vi "Build Spec Param to XPath.vi"(0 "NI Build Specification":refnum<class "NI Build Specification_LV.lvclass">, 5 "Build Spec Parameter Name":string, 11 "error in (no error)":errorcluster) -> (4 "NI Build Specification":refnum<class "NI Build Specification_LV.lvclass">, 6 "XPath to the specific build Spec Property":string, 15 "error out":errorcluster)   [LabVIEW 2017, in "CL_G3_VIComponentBuilder.lvlib" / "NI Build Specification_LV.lvclass"]
doc: "Returns an Xpath to the parameter of a build specification."
uses:
  NI Build Specification_LV.lvclass
  NI Build Specification_LV.lvclass/NI Build Specification_LV.ctl
  Accessors/Read Target Name Containing Build Specs to Build.vi
  Accessors/Read Export's Build Spec Name.vi
  Accessors/Read Build Spec Type.vi
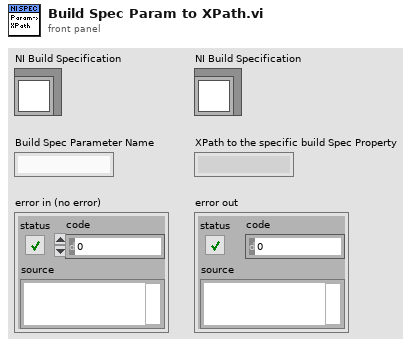
[diagram p1: front panel]
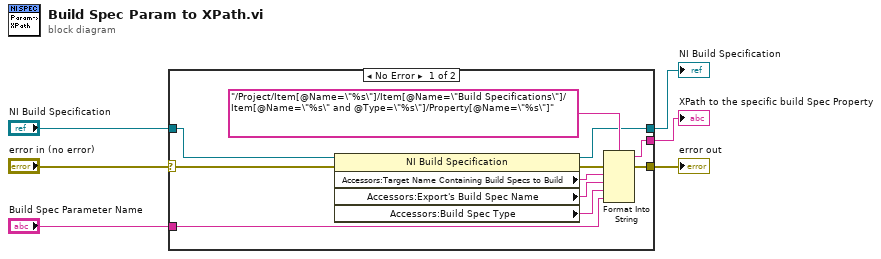
[diagram p0: block diagram]
diagram:
  n1 = case shown="No Error" "error in (no error)" {
    selector: "error in (no error)" -> [w8 w18]
    tunnel: "NI Build Specification" -> [w17 w19]
    tunnel: [w15 w19] -> w5
    tunnel: [w11 _] -> w4
    tunnel: "Build Spec Parameter Name" -> [w9 _]
    tunnel: [w7 w18] -> w1
    frame No Error {
      n2 = property class="NI Build Specification"(reference=w17, error in=w8) -> (reference out=w15:refnum<class "NI Build Specification_LV.lvclass">, error out=w10:errorcluster, "Accessors:Target Name Containing Build Specs to Build"=w14:string, "Accessors:Export's Build Spec Name"=w13:string, "Accessors:Build Spec Type"=w12:string)
      n3 = Format Into String(format string="/Project/Item[@Name=\"%s\"]/Item[@Name=\"Build Specifications\"]/Item[@Name=\"%s\" and @Type=\"%s\"]/Property[@Name=\"%s\"]", error in=w10, w14, w13, w12, w9) -> (resulting string=w11:string, error out=w7:errorcluster)  [unwired: 1 in]
    }
    frame Error {
    }
  }
  "XPath to the specific build Spec Property" <- w4
  "NI Build Specification" <- w5
  "error out" <- w1
